vi "macierz i wyznacznik.vi"() -> ()   [LabVIEW 2020]
uses:
  <vilib>/Analysis/baseanly.llb/Real Determinant.vi
  <vilib>/Analysis/NI_AALBase.lvlib
panel:
  out "Wyznacznik":dbl format="%.2e"
  out "Usunieta kolumna":dbl[](array[numeric])
  out "Usunieta kolumna jako wiersz":dbl[](array[numeric])
  out "Tablica bez ostatniej kolumny":dbl[][](array[numeric])
  in  "Pierwsza tablica":dbl[][](array[numeric])
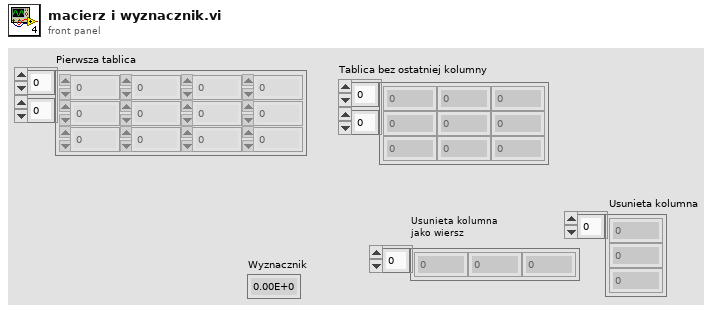
[diagram p1: front panel]
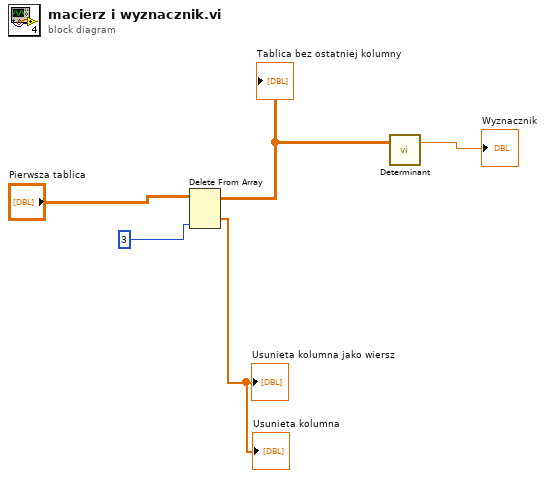
[diagram p0: block diagram]
diagram:
  n1 = Delete From Array(array="Pierwsza tablica", index (col)=3) -> (deleted portion=→"Usunieta kolumna jako wiersz" →"Usunieta kolumna":dbl[], array with subset deleted=w2:dbl[][])  [unwired: 2 in]
  "Tablica bez ostatniej kolumny" <- w2
  n2 = call-poly <vilib>:"Determinant.vi"("Input Matrix"=w2) -> ("determinant"=→"Wyznacznik":dbl)  [unwired: 1 in, 1 out]
